vi "readBackGround.vi"(8 "error in (no error)":errorcluster, 11 "file (use dialog)":path) -> (0 "error out":errorcluster, 3 "initialized array":sgl[][](array[numeric]) format="%.2f")   [LabVIEW 2020]
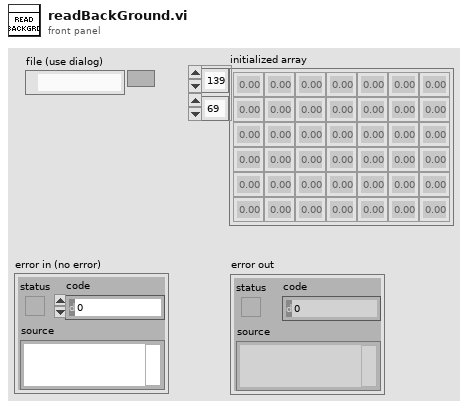
[diagram p1: front panel]
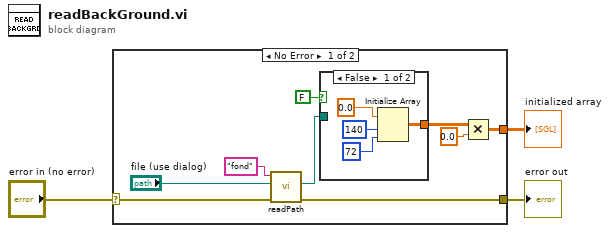
[diagram p0: block diagram]
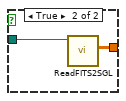
[diagram p2: hidden frame]
diagram:
  n1 = case shown="No Error" "error in (no error)" {
    selector: "error in (no error)" -> [w6 w19]
    tunnel: [w5 _] -> w3
    tunnel: [w7 w19] -> w2
    frame No Error {
      n2 = call "readPath.vi"("error in (no error)"=w6, "file (use dialog)"="file (use dialog)", "regular expression"="fond") -> ("error out"=w7:errorcluster, "path"=w11:path)  [unwired: 6 in, 1 out]
      n3 = case shown="False" FALSE {
        tunnel: w11 -> [_ w18]
        tunnel: [w16 w17] -> w9
        frame False {
          n4 = Initialize Array(sgl 0.0 ("element"), 140 ("dimension size"), 72 ("dimension size")) -> (w16:sgl[][])
        }
        frame True {
          n5 = call "ReadFITS2SGL.vi"("Path"=w18) -> ("Tableau2DSGL"=w17:sgl[][])  [unwired: 7 in, 3 out]
        }
      }
      n6 = Multiply(x=w9, y=sgl 0.0) -> (x*y=w5:sgl[][])
    }
    frame Error {
    }
  }
  "initialized array" <- w3
  "error out" <- w2
